vi "SigSyn-Create (polymorphic).vi"   [LabVIEW 2020]
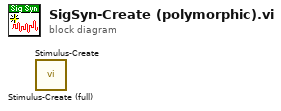
[diagram p0: block diagram]
diagram:
  n1 = call "Stimulus-Create (full).vi"() -> ()  [unwired: 8 in, 4 out]
  n2 = call "Stimulus-Create.vi"() -> ()  [unwired: 8 in, 4 out]
